vi "Debug Exercise (Sub).vi"(1 "Number":dbl format="%.2f") -> (0 "Final Result":dbl format="%.2f")   [LabVIEW 2019]
doc: "This VI is the subVI for Exercise 2-3 of the LabVIEW Basics I Course."
panel:
  in  "Stop Button":bool
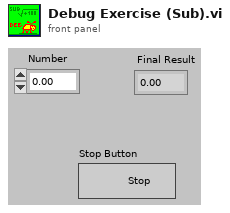
[diagram p1: front panel]
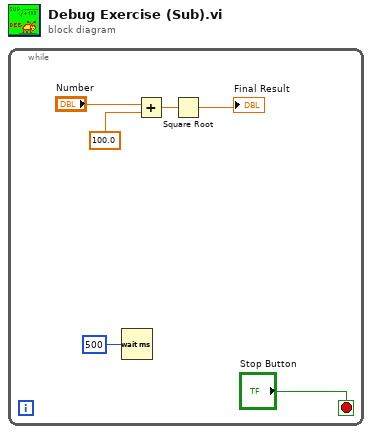
[diagram p0: block diagram]
diagram:
  n1 = while {
    stop <- "Stop Button" stop-if-true
    n2 = Wait (ms)(milliseconds to wait=u32 500 ("millisecond timer value")) -> ()  [unwired: 1 out]
    n3 = Add(x="Number", y=100.0) -> (x+y=w3:dbl)
    n4 = Square Root(x=w3) -> (sqrt(x)=→"Final Result":dbl)
  }
